vi "boolean2string.vi"(1 "Boolean":bool) -> (0 "String":string)   [LabVIEW 2021]
doc: "This VI converts a boolean to a string.\nResult is either True or False."
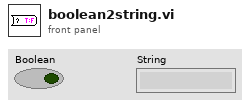
[diagram p1: front panel]
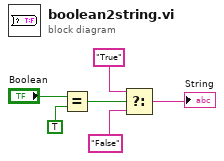
[diagram p0: block diagram]
diagram:
  n1 = Equal?(x="Boolean", y=TRUE) -> (x = y?=w5:bool)
  n2 = Select(t="True", s=w5, f="False") -> (s? t:f=→"String":string)
